vi "ConfigInstr.vi"(6 "InstrumentName":string, 7 "VisaRessIn":refnum<visa-resource-name>, 8 "error in (no error)":errorcluster caption="entrée d'erreur (pas d'erreur)", 9 "FirstClassInst":bool, 10 "Function":string, 11 "Device en entrée":refnum<class "BaseDevice.lvclass"> caption="DNL_LabVIEW Object in") -> (0 "error out":errorcluster caption="sortie d'erreur", 3 "Device en sortie":refnum<class "BaseDevice.lvclass"> caption="DNL_LabVIEW Object out")   [LabVIEW 2019, in "BaseDevice.lvclass"]
uses:
  BaseDevice.lvclass
  BaseDevice_Func.ctl
  BaseDevice.lvclass/BaseDevice.ctl
panel:
  out "VisaRessOut":refnum<visa-resource-name>
  in  "Dev_Func":T1
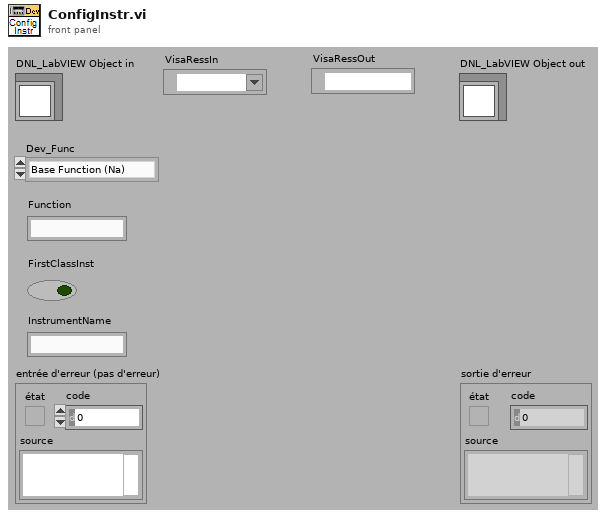
[diagram p1: front panel]
types:
  T1 = typedef "BaseDevice.lvclass/BaseDevice_Func.ctl" = enum16{"Base Function (Na)"}
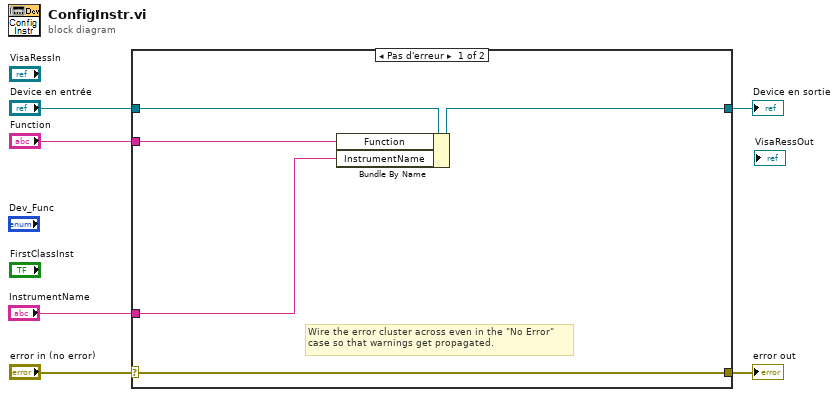
[diagram p0: block diagram]
diagram:
  n1 = case shown="Pas d'erreur" "error in (no error)" {
    selector: "error in (no error)" -> [w11 w13]
    tunnel: [w11 w13] -> w5
    tunnel: [w9 w12] -> w3
    tunnel: "Device en entrée" -> [w10 w12]
    tunnel: "Function" -> [w7 _]
    tunnel: "InstrumentName" -> [w8 _]
    frame No Error {
      # "Wire the error cluster across even in the \"No Error\"\ncase so that warnings get propagated."
      n2 = Bundle By Name(cluster=w10, "Function"=w7, "InstrumentName"=w8) -> (w9:refnum<class "BaseDevice.lvclass">)
    }
    frame Error {
    }
  }
  "error out" <- w5
  "Device en sortie" <- w3
